vi "Serial Write to DB.vi"(6 "Chamber ID":T2(array[cluster])=[{"Chamber name"="Analysis", "Trip pressure"=5e-07}, {"Chamber name"="Prep", "Trip pressure"=3e-05}], 8 "error in (no error) 2":errorcluster, 9 "Trip Pressures 2":dbl[](array[numeric]), 10 "AML Cluster const":T1[](array[typedef]), 11 "Data.PG in":refnum<class "LV-Data.PGSQL.lvclass">) -> (0 "error in (no error)":errorcluster, 1 "Paths":string[](array[string]), 2 "Successful Writes":bool[](array[boolean]), 3 "Data.PG out":refnum<class "LV-Data.PGSQL.lvclass">)   [LabVIEW 2019]
uses:
  <userlib>/LevyLab/LV-Data/LV-Data.PG/LV-Data.PGSQL.lvclass
  Labview clones/AML-UHV-Gauge-Controller/lvsrc/sandbox/Instrument.AML.GetAll--Cluster.ctl
  <userlib>/LevyLab/LV-Data/LV-Data.PG/API/Write Variable (one-row).vi
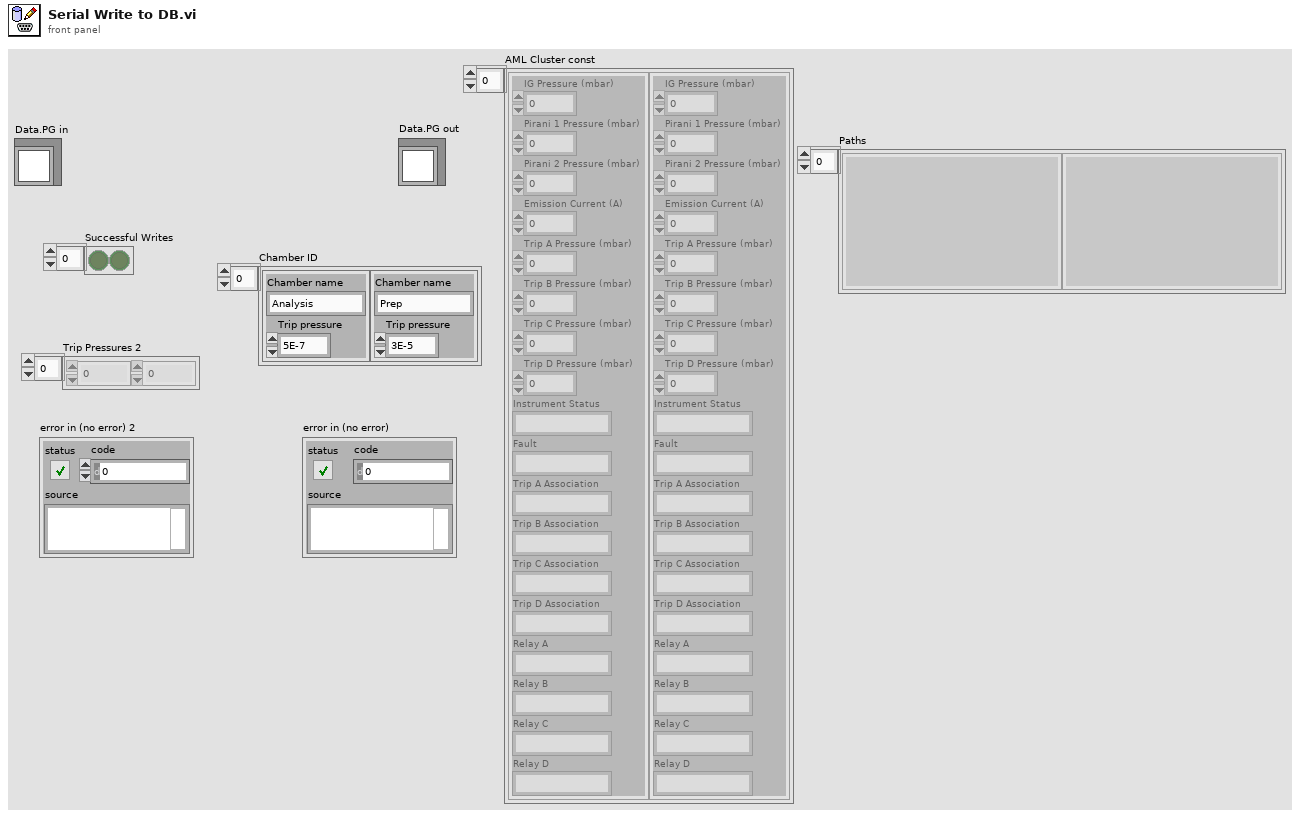
[diagram p1: front panel]
types:
  T1 = typedef "Instrument.AML.GetAll--Cluster.ctl" = cluster{"IG Pressure (mbar)":dbl, "Pirani 1 Pressure (mbar)":dbl, "Pirani 2 Pressure (mbar)":dbl, "Emission Current (A)":dbl, "Trip A Pressure (mbar)":dbl, "Trip B Pressure (mbar)":dbl, "Trip C Pressure (mbar)":dbl, "Trip D Pressure (mbar)":dbl, "Instrument Status":string, "Fault":string, "Trip A Association":string, "Trip B Association":string, "Trip C Association":string, "Trip D Association":string, "Relay A":string, "Relay B":string, "Relay C":string, "Relay D":string}
  T2 = cluster{"Chamber name":string, "Trip pressure":dbl}[]
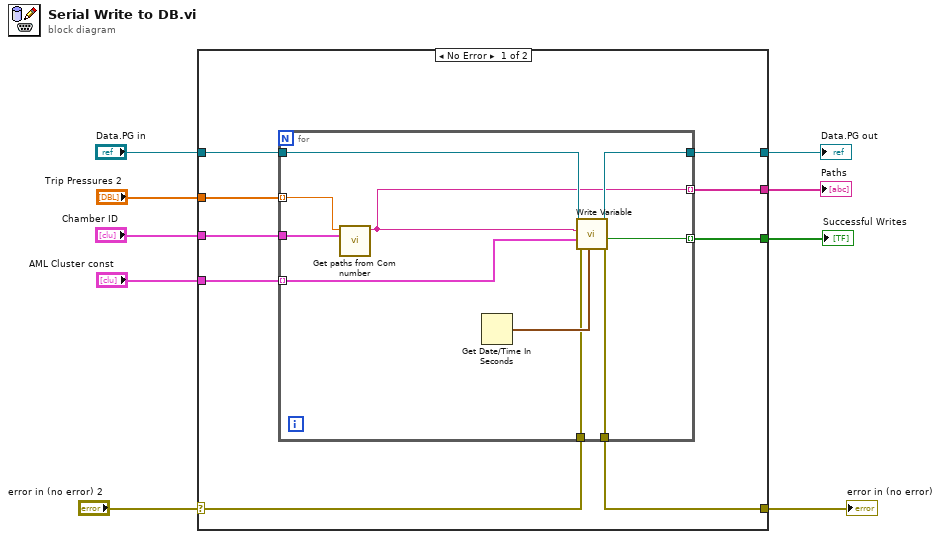
[diagram p0: block diagram]
diagram:
  n1 = case shown="No Error" "error in (no error) 2" {
    selector: "error in (no error) 2" -> [w18 w30]
    tunnel: [w17 w30] -> w8
    tunnel: "Data.PG in" -> [w16 w29]
    tunnel: [w15 w29] -> w6
    tunnel: [w14 _] -> w5
    tunnel: "AML Cluster const" -> [w13 _]
    tunnel: "Chamber ID" -> [w12 _]
    tunnel: "Trip Pressures 2" -> [w11 _]
    tunnel: [w10 _] -> w1
    frame No Error {
      n2 = for {
        tunnel: w18 -> [w27]
        tunnel: [w26] -> w17
        tunnel: w16 -> [w25]
        tunnel: [w24] -> w15
        tunnel: [w23] -> w14 mode=indexing
        tunnel: w13 -> [w22] mode=indexing
        tunnel: w12 -> [w21]
        tunnel: w11 -> [w19] mode=indexing
        tunnel: [w20] -> w10 mode=indexing
        n3 = call "Get paths from Com number.vi"("Chamber ID"=w21, "Trip pressure"=w19) -> ("String"=w20:string)  [unwired: 9 in]
        n4 = Get Date/Time In Seconds() -> (seconds since 1Jan1904=w28:timestamp)
        n5 = call-poly <userlib>:"Write Variable.vi"("Time Stamp"=w28, "error in (no error)"=w27, "Data"=w22, "variable"=w20, "Data.PG in"=w25) -> ("error out"=w26:errorcluster, "Wrote to DB?"=w23:bool, "Data.PG out"=w24:refnum<class "LV-Data.PGSQL.lvclass">)  [unwired: 3 in, 1 out]
      }
    }
    frame Error {
    }
  }
  "error in (no error)" <- w8
  "Data.PG out" <- w6
  "Successful Writes" <- w5
  "Paths" <- w1
